vi "Z010生成条码.vi"(2 "产品ID":string, 3 "芯片编码":string) -> ()   [LabVIEW 2013]
uses:
  <vilib>/Utility/error.llb/whitespace.ctl
panel:
  in  "error in (no error)":errorcluster
  out "error out":errorcluster
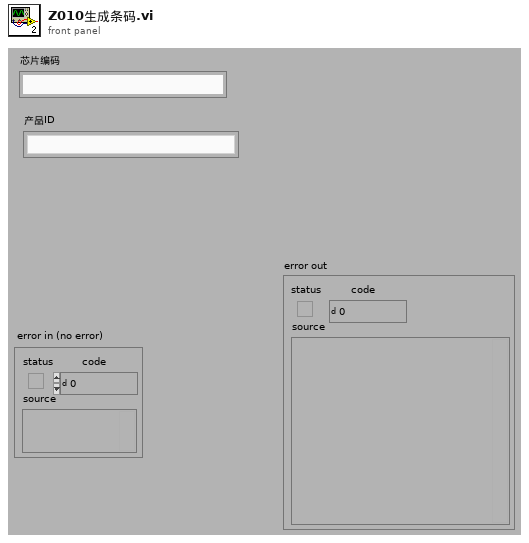
[diagram p1: front panel]
types:
  T1 = typedef "whitespace.ctl" = u16
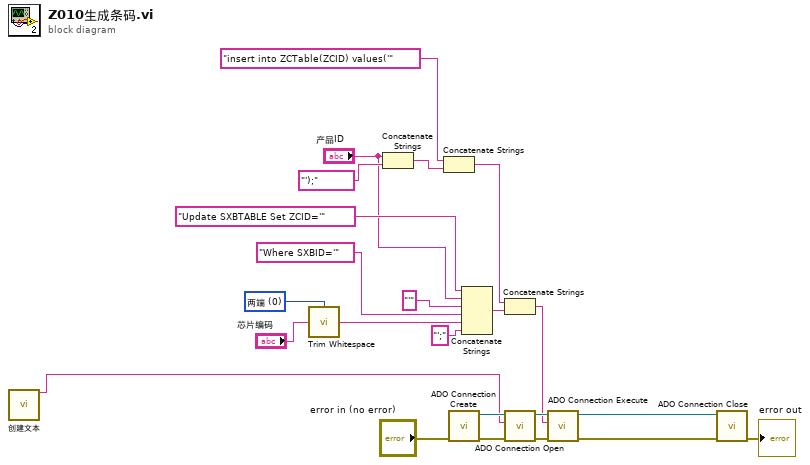
[diagram p0: block diagram]
diagram:
  w10 = T1 0 items=["两端", "字符串首端", "字符串末端"] ("location (both)")
  n1 = call "创建文本"() -> ("Result"=w1:string)  [unwired: 14 in, 1 out]
  n2 = call <vilib>:"Trim Whitespace.vi"("string"="芯片编码", "location (both)"=w10) -> ("trimmed string"=w8:string)
  n3 = Concatenate Strings("产品ID", "');" ("字符串")) -> (w11:string)
  n4 = Concatenate Strings("insert into ZCTable(ZCID) values('" ("字符串"), w11) -> (w13:string)
  n5 = call "ADO Connection Create.vi"("error in (no error)"="error in (no error)") -> ("error out"=w22:errorcluster, "ADODB._Connection Out"=w23:refnum<k7>)  [unwired: 9 out]
  n6 = Concatenate Strings("Update SXBTABLE Set ZCID='" ("字符串"), "产品ID", "'" ("字符串"), "Where SXBID='" ("字符串"), w8, "';" ("字符串")) -> (w3:string)
  n7 = Concatenate Strings(w13, w3) -> (w12:string)
  n8 = call "ADO Connection Open.vi"("error in (no error)"=w22, "ConnectionString"=w1, "ADODB._Connection In"=w23) -> ("error out"=w21:errorcluster, "ADODB._Connection Out"=w20:refnum<k7>)  [unwired: 7 out]
  n9 = call "ADO Connection Execute.vi"("error in (no error)"=w21, "CommandText"=w12, "ADODB._Connection In"=w20) -> ("error out"=w15:errorcluster, "ADODB._Connection Out"=w19:refnum<k7>)  [unwired: 7 out]
  n10 = call "ADO Connection Close.vi"("error in (no error)"=w15, "ADODB._Connection In"=w19) -> ("error out"=→"error out":errorcluster)  [unwired: 9 out]
